vi "Control-Script-Host.vi"() -> ()   [LabVIEW 2016]
uses:
  <vilib>/gmath/NI_Gmath.lvlib
panel:
  out "Error":bool caption="RT Error"
  out "_Syntax Error":bool caption="Syntax Error"
  out "Channels":T1(array[cluster])
  in  "Enable":bool
  out "In Variable":cluster{"Name":string}[](array[cluster])
  in  "Script":string
  in  "Parsed":T2 {"Y Values" format="%.2f"}
  out "Out Variable":cluster{"Name":string}[](array[cluster])
  in  "Outputs":T1(array[cluster])
  # "User Script (Control)"
  # "operator"
  # "register1"
  # "register2"
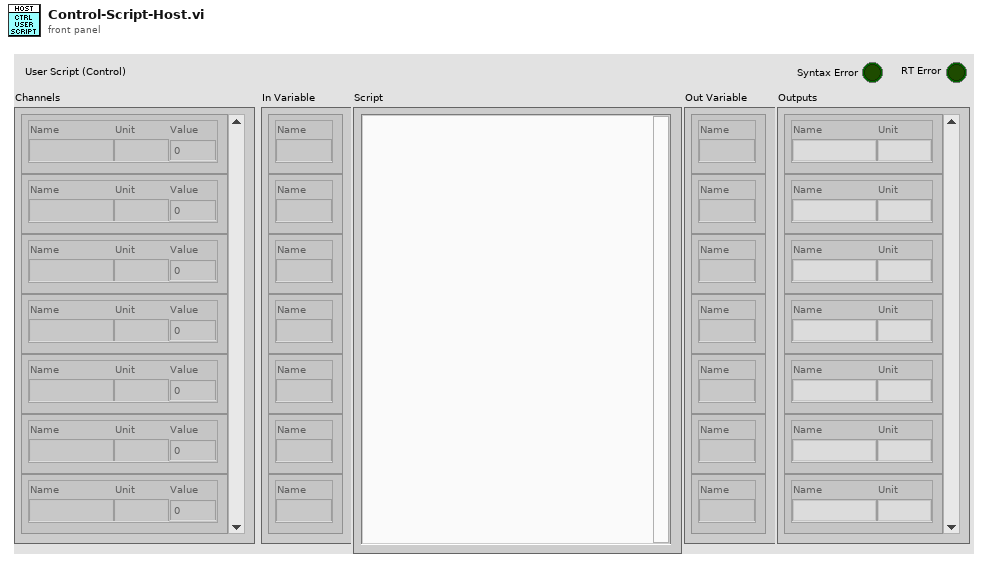
[diagram p1: front panel]
types:
  T1 = cluster{"Name":string, "Unit":string, "Value":dbl}[]
  T2 = cluster{"Y Values":dbl[][], "Tables":i32[][][], "Variables input decode":i32[], "Variables output decode":i32[]}
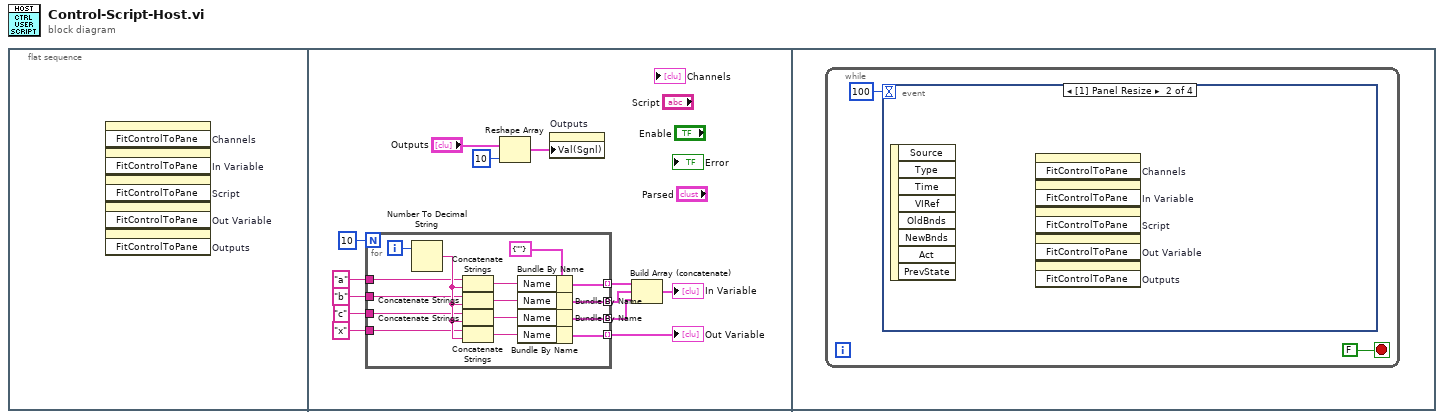
[diagram p0: block diagram]
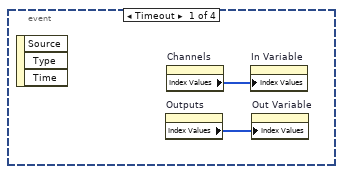
[diagram p2: hidden frame]
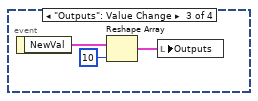
[diagram p3: hidden frame]
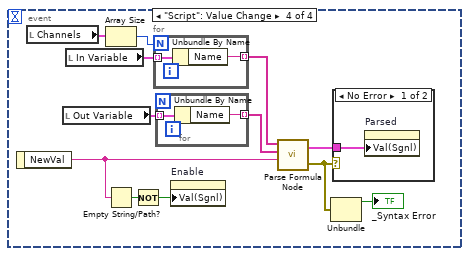
[diagram p4: hidden frame]
diagram:
  n1 = flat-sequence {
    frame #0 {
      n2 = invoke on="Channels" class="Arr (strict)" method="FitControlToPane"() -> ()  [unwired: 3 in, 3 out]
      n3 = invoke on="In Variable" class="Arr (strict)" method="FitControlToPane"() -> ()  [unwired: 3 in, 3 out]
      n4 = invoke on="Script" class="Str" method="FitControlToPane"() -> ()  [unwired: 3 in, 3 out]
      n5 = invoke on="Out Variable" class="Arr (strict)" method="FitControlToPane"() -> ()  [unwired: 3 in, 3 out]
      n6 = invoke on="Outputs" class="Arr (strict)" method="FitControlToPane"() -> ()  [unwired: 3 in, 3 out]
    }
    frame #1 {
      n7 = for {
        N: 10 -> [_]
        tunnel: "a" -> [w23]
        tunnel: "b" -> [w24]
        tunnel: "c" -> [w25]
        tunnel: "x" -> [w26]
        tunnel: [w14] -> w8 mode=indexing
        tunnel: [w15] -> w7 mode=indexing
        tunnel: [w16] -> w6 mode=indexing
        tunnel: [w17] -> w5 mode=indexing
        i -> [w28]
        w21 = cluster{"Name":string} {"Name"=""} ("Cluster")
        n8 = Number To Decimal String(number=w28) -> (decimal integer string=w27:string)  [unwired: 1 in]
        n9 = Concatenate Strings(w23, w27) -> (w22:string)
        n10 = Concatenate Strings(w24, w27) -> (w20:string)
        n11 = Concatenate Strings(w25, w27) -> (w19:string)
        n12 = Concatenate Strings(w26, w27) -> (w18:string)
        n13 = Bundle By Name(cluster=w21, "Name"=w22) -> (w14:cluster{"Name":string})
        n14 = Bundle By Name(cluster=w21, "Name"=w20) -> (w15:cluster{"Name":string})
        n15 = Bundle By Name(cluster=w21, "Name"=w19) -> (w16:cluster{"Name":string})
        n16 = Bundle By Name(cluster=w21, "Name"=w18) -> (w17:cluster{"Name":string})
      }
      "Out Variable" <- w5
      n17 = Reshape Array("Outputs", 10 ("dimension size")) -> (w1:T1)
      n18 = property on="Outputs" class="Arr (strict)"("Val(Sgnl)"=w1) -> ()  [unwired: 2 in, 2 out]
      n19 = Build Array (concatenate)(w8, w7, w6) -> (→"In Variable":cluster{"Name":string}[])
    }
    frame #2 {
      n20 = while {
        stop <- FALSE stop-if-true
        n21 = event shown="[1] Panel Resize" {
          selector: _ -> [_ _ _ _]
          dyn-events: _ -> [_ _ _ _]
          timeout: 100 -> [_ _ _ _]
          event Timeout {
            n22 = event-data() -> ()  [unwired: 1 in, 3 out]
            n23 = property on="Outputs" class="Arr (strict)"() -> ("Index Values"=w31:u32[])  [unwired: 2 in, 2 out]
            n24 = property on="Channels" class="Arr (strict)"() -> ("Index Values"=w32:u32[])  [unwired: 2 in, 2 out]
            n25 = property on="In Variable" class="Arr (strict)"("Index Values"=w32) -> ()  [unwired: 2 in, 2 out]
            n26 = property on="Out Variable" class="Arr (strict)"("Index Values"=w31) -> ()  [unwired: 2 in, 2 out]
          }
          event Panel Resize {
            n27 = event-data() -> ()  [unwired: 1 in, 8 out]
            n28 = invoke on="Channels" class="Arr (strict)" method="FitControlToPane"() -> ()  [unwired: 3 in, 3 out]
            n29 = invoke on="In Variable" class="Arr (strict)" method="FitControlToPane"() -> ()  [unwired: 3 in, 3 out]
            n30 = invoke on="Script" class="Str" method="FitControlToPane"() -> ()  [unwired: 3 in, 3 out]
            n31 = invoke on="Out Variable" class="Arr (strict)" method="FitControlToPane"() -> ()  [unwired: 3 in, 3 out]
            n32 = invoke on="Outputs" class="Arr (strict)" method="FitControlToPane"() -> ()  [unwired: 3 in, 3 out]
          }
          event "Outputs": Value Change {
            n33 = event-data() -> ("NewVal"=w35:T1)  [unwired: 1 in]
            n34 = Reshape Array(w35, 10 ("dimension size")) -> (w33:T1)
            n35 = local write "Outputs"(w33) -> ()
          }
          event "Script": Value Change {
            n36 = event-data() -> ("NewVal"=w38:string)  [unwired: 1 in]
            n37 = local read "Channels"() -> (w40:T1)
            n38 = local read "Out Variable"() -> (w47:cluster{"Name":string}[])
            n39 = local read "In Variable"() -> (w45:cluster{"Name":string}[])
            n40 = Array Size(array=w40) -> (size(s)=w39:i32)
            n41 = Empty String/Path?(string/path=w38) -> (empty?=w37:bool)
            n42 = Not(x=w37) -> (.not. x?=w36:bool)
            n43 = for {
              N: w39 -> [_]
              tunnel: w45 -> [w49] mode=indexing
              tunnel: [w48] -> w44 mode=indexing
              n44 = Unbundle By Name(w49) -> ("Name"=w48:string)
            }
            n45 = for {
              tunnel: w47 -> [w51] mode=indexing
              tunnel: [w50] -> w46 mode=indexing
              n46 = Unbundle By Name(w51) -> ("Name"=w50:string)
            }
            n47 = property on="Enable" class="Bool (strict)"("Val(Sgnl)"=w36) -> ()  [unwired: 2 in, 2 out]
            n48 = call <vilib>:"Parse Formula Node.vi"("formula"=w38, "Variables Output"=w46, "Variables Input"=w44) -> ("error out"=w41:errorcluster, "Parsed Formula Node"=w42:T2)  [unwired: 1 in]
            n49 = Unbundle(w41) -> ("status"=→"_Syntax Error":bool)  [unwired: 2 out]
            n50 = case shown="No Error" w41 {
              tunnel: w42 -> [w52 _]
              frame No Error {
                n51 = property on="Parsed" class="Clust (strict)"("Val(Sgnl)"=w52) -> ()  [unwired: 2 in, 2 out]
              }
              frame Error {
              }
            }
          }
        }
      }
    }
  }
